vi "Initialize Weather Station.vi"(8 "에러 입력(에러 없음)":errorcluster) -> (0 "에러 출력":errorcluster, 3 "파일 참조 번호":refnum<file>, 5 "날씨 데이터":T1)   [LabVIEW 2010]
doc: "이 VI는 기상 관측기 프로젝트의 일부입니다.날씨 데이터 클러스터와 텍스트 파일(Weather.txt)이 생성되었습니다. 날씨 데이터 클러스터를 나타내는 머리글이 파일에 작성되었습니다. \n\n입력: 에러 입력\n출력: 파일 참조 번호, 날씨 데이터 클러스터, 에러 출력"
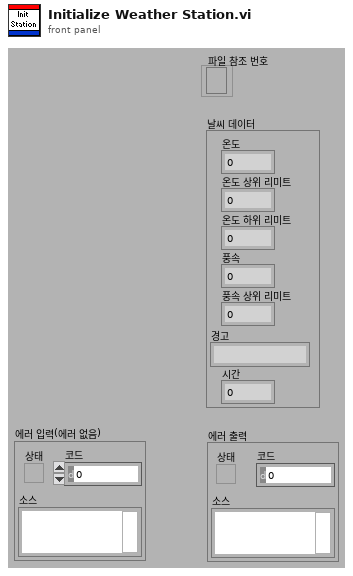
[diagram p1: front panel]
types:
  T1 = cluster{"온도":dbl, "온도 상위 리미트":dbl, "온도 하위 리미트":dbl, "풍속":dbl, "풍속 상위 리미트":dbl, "경고":string, "시간":dbl}
  T2 = enum16{"open", "replace", "create", "open or create", "replace or create", "replace or create with confirmation"}
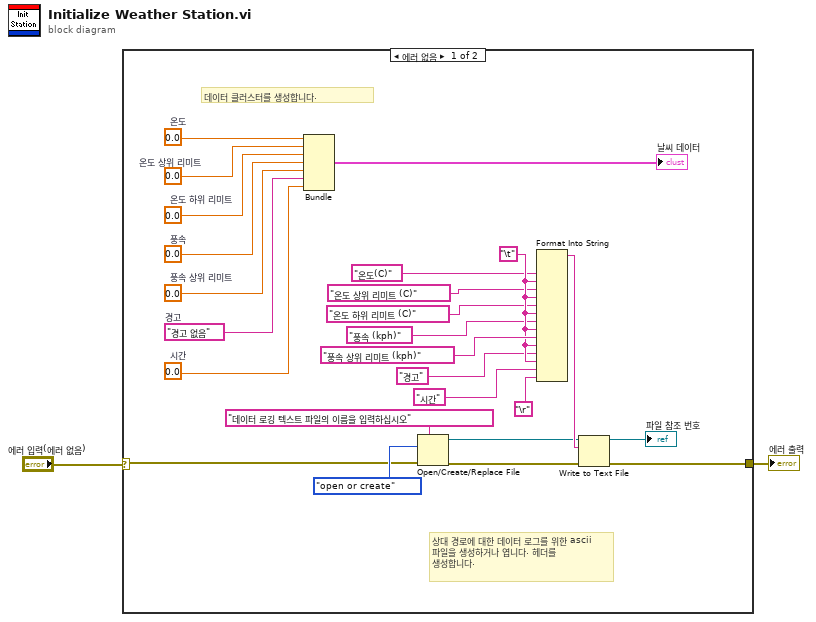
[diagram p0: block diagram]
diagram:
  n1 = case shown="에러 없음" "에러 입력(에러 없음)" {
    selector: "에러 입력(에러 없음)" -> [w4 w28]
    tunnel: [w26 w28] -> w2
    frame No Error {
      w12 = 0.0  # 시간
      w11 = 0.0  # 풍속 상위 리미트
      w10 = 0.0  # 풍속
      w5 = 0.0  # 온도 하위 리미트
      w6 = 0.0  # 온도 상위 리미트
      w7 = 0.0  # 온도
      w20 = "\t"
      w9 = "경고 없음"  # 경고
      # "상대 경로에 대한 데이터 로그를 위한 ascii 파일을 생성하거나 엽니다. 헤더를 생성합니다."
      # "데이터 클러스터를 생성합니다."
      n2 = Bundle("온도"=w7, "온도 상위 리미트"=w6, "온도 하위 리미트"=w5, "풍속"=w10, "풍속 상위 리미트"=w11, "경고"=w9, "시간"=w12) -> (→"날씨 데이터":T1)  [unwired: 1 in]
      n3 = Open/Create/Replace File(error in=w4, prompt="데이터 로깅 텍스트 파일의 이름을 입력하십시오", operation (0:open)=T2."open or create") -> (refnum out=w23:refnum<file>, error out=w25:errorcluster)  [unwired: 3 in, 1 out]
      n4 = Format Into String("온도(C)", w20, "온도 상위 리미트 (C)", w20, "온도 하위 리미트 (C)", w20, "풍속 (kph)", w20, "풍속 상위 리미트 (kph)", w20, "경고", w20, "시간", "\r") -> (resulting string=w27:string)  [unwired: 3 in, 1 out]
      n5 = Write to Text File(file (use dialog)=w23, text=w27, error in=w25) -> (refnum out=→"파일 참조 번호":refnum<file>, error out=w26:errorcluster)  [unwired: 1 in, 1 out]
    }
    frame Error {
    }
  }
  "에러 출력" <- w2
